vi "Move or Copy Element.vi"(8 "error in (no error)":errorcluster, 10 "Move or Copy Element":T1, 11 "Test Executive Builder Model in":refnum<class "Test Executive Builder Model.lvclass">) -> (0 "error out":errorcluster, 3 "Test Executive Builder Model out":refnum<class "Test Executive Builder Model.lvclass">, 5 "Unique ID":string)   [LabVIEW 2017, in "Test Executive Builder Model.lvclass"]
uses:
  Test Executive Builder Model.lvclass
  <vilib>/gpm_packages/@cs/test-executive/Source/Test Executive/TestExecutive Ref/TestExecutive Ref.lvclass
  Test Executive Builder Model Messages/Redraw Tree Msg/Redraw Tree Msg.lvclass
  <vilib>/ActorFramework/Actor/Actor.lvclass
  C:/Program Files (x86)/National Instruments/LabVIEW 2017/vi.lib/ActorFramework/Actor/Actor.lvclass
  Application Dependencies/Move or Copy Element.ctl
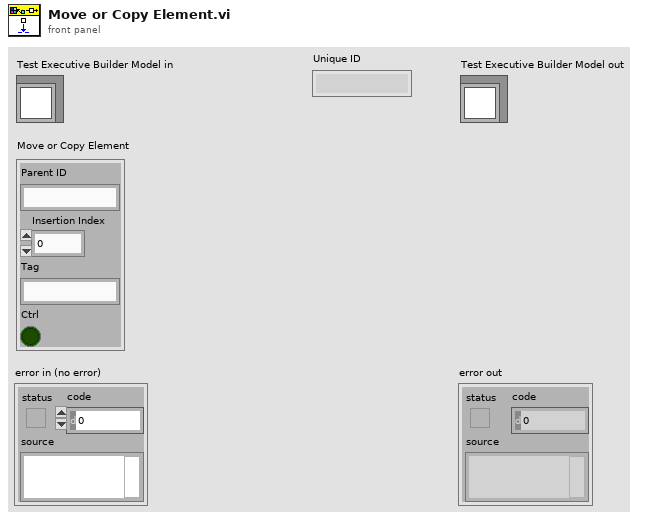
[diagram p1: front panel]
types:
  T1 = typedef "Move or Copy Element.ctl" = cluster{"Parent ID":string, "Insertion Index":i32, "Tag":string, "Ctrl":bool}
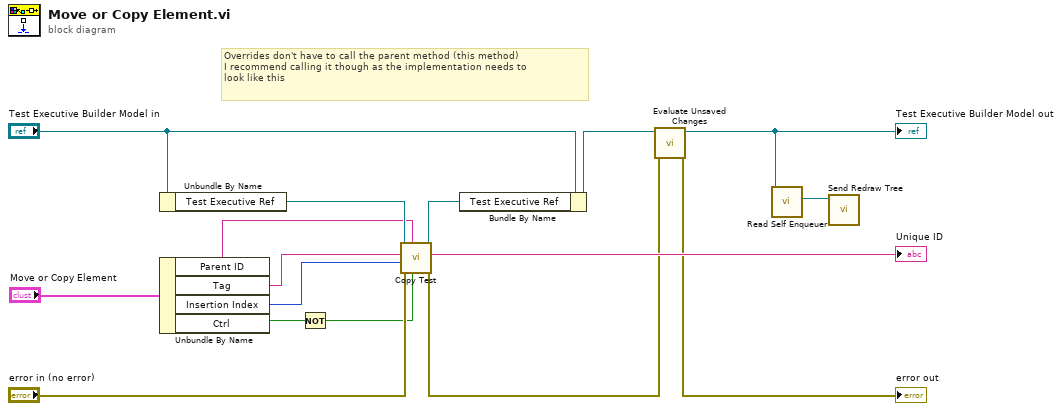
[diagram p0: block diagram]
diagram:
  # "Overrides don't have to call the parent method (this method)\nI recommend calling it though as the implementation needs to\nlook like this"
  n1 = Unbundle By Name("Test Executive Builder Model in") -> ("Test Executive Ref"=w16:refnum<data-value>)
  n2 = Unbundle By Name("Move or Copy Element") -> ("Parent ID"=w11:string, "Tag"=w10:string, "Insertion Index"=w9:i32, "Ctrl"=w8:bool)
  n3 = Not(x=w8) -> (.not. x?=w7:bool)
  n4 = call <vilib>:"Copy Test.vi"("Move?"=w7, "New Parent ID"=w11, "error in (no error)"="error in (no error)", "Insertion Index"=w9, "Test ID"=w10, "Test Executive Ref"=w16) -> ("error out"=w2:errorcluster, "Test ID out"=→"Unique ID":string, "Test Executive Ref out"=w14:refnum<data-value>)  [unwired: 3 in]
  n5 = Bundle By Name(cluster="Test Executive Builder Model in", "Test Executive Ref"=w14) -> (w4:refnum<class "Test Executive Builder Model.lvclass">)
  n6 = call-dynamic "Evaluate Unsaved Changes.vi"("error in (no error)"=w2, "Test Executive Builder Model in"=w4) -> ("error out"=→"error out":errorcluster, "Test Executive Builder Model out"=w3:refnum<class "Test Executive Builder Model.lvclass">)  [unwired: 8 in]
  "Test Executive Builder Model out" <- w3
  n7 = call <vilib>:"Read Self Enqueuer.vi"("Actor"=w3) -> ("Self Enqueuer"=w5:refnum<class "Message Enqueuer.lvclass">)  [unwired: 10 in]
  n8 = call "Send Redraw Tree.vi"("Message Enqueuer"=w5) -> ()  [unwired: 9 in, 2 out]
